vi "Table Heading Cell.vi"(4 "Class (\"\")":string, 6 "Cell Heading String (\"\")":string, 7 "Previous HTML in":string) -> (3 "HTML out":string)   [LabVIEW 2011]
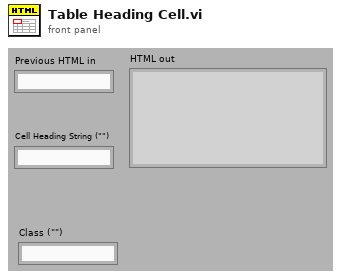
[diagram p1: front panel]
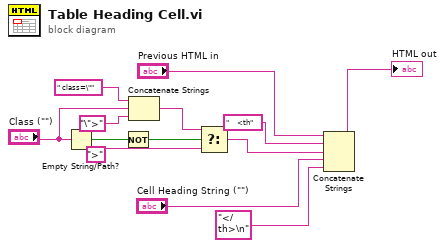
[diagram p0: block diagram]
diagram:
  n1 = Empty String/Path?(string/path="Class (\"\")") -> (empty?=w8:bool)
  n2 = Not(x=w8) -> (.not. x?=w4:bool)
  n3 = Concatenate Strings(" class=\"", "Class (\"\")", "\">") -> (w6:string)
  n4 = Select(t=w6, s=w4, f=">") -> (s? t:f=w1:string)
  n5 = Concatenate Strings("Previous HTML in", "    <th", w1, "Cell Heading String (\"\")", "</th>\n") -> (→"HTML out":string)
